vi "Export Steering Frame to VI.vi"(8 "error in (no error)":errorcluster, 10 "vi path":path, 11 "steering frame in":refnum<class "NI_Robotics_Steering Frame.lvclass">) -> (0 "error out":errorcluster, 3 "steering frame out":refnum<class "NI_Robotics_Steering Frame.lvclass">)   [LabVIEW 2017, in "NI_Robotics_Configure Steering Frame.lvlib"]
uses:
  <vilib>/robotics/Dialog/Configure Steering Frame/NI_Robotics_Configure Steering Frame.lvlib
  <vilib>/robotics/Steering/Steering Frame/NI_Robotics_Steering Frame.lvclass
  <vilib>/robotics/Utilities/Scripting/NI_Robotics_Scripting Utilities.lvlib
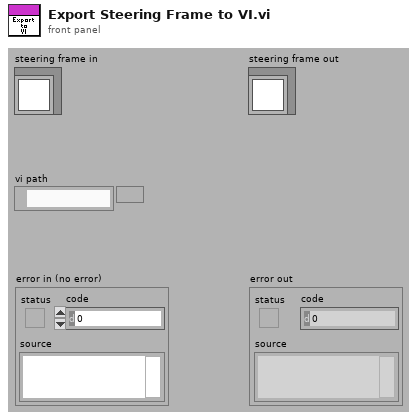
[diagram p1: front panel]
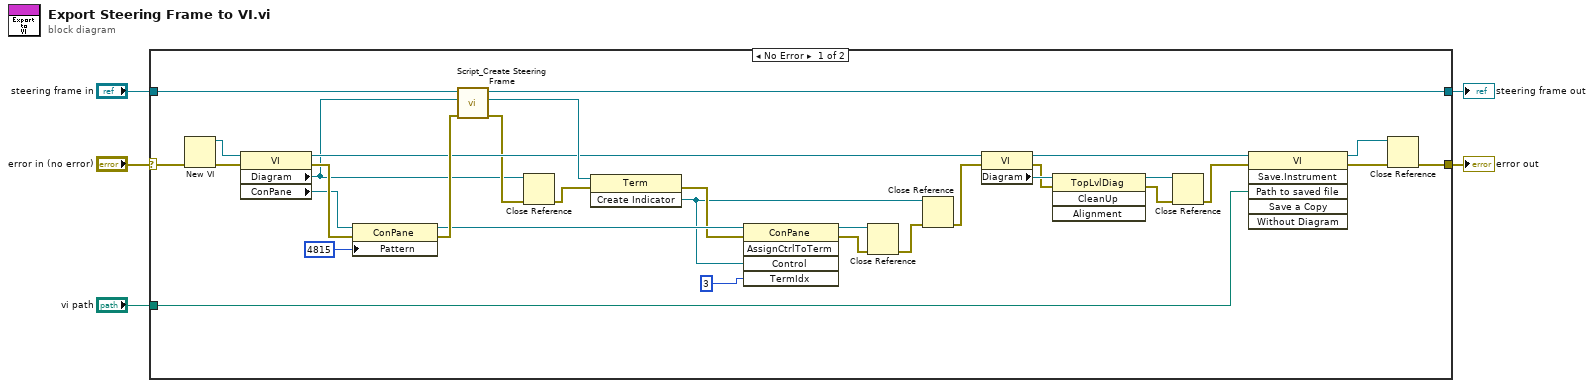
[diagram p0: block diagram]
diagram:
  n1 = case shown="No Error" "error in (no error)" {
    selector: "error in (no error)" -> [w37 w38]
    tunnel: "steering frame in" -> [w36 w39]
    tunnel: "vi path" -> [w21 _]
    tunnel: [w35 w39] -> w2
    tunnel: [w19 w38] -> w1
    frame No Error {
      n2 = New VI(8:w37) -> (0:w32:errorcluster, 3:w33:refnum<vi>)  [unwired: 6 in]
      n3 = property class="VI"(reference=w33, error in=w32) -> (reference out=w16:refnum<vi>, error out=w30:errorcluster, "Diagram"=w7:refnum<vi>, "ConPane"=w9:refnum<vi>)
      n4 = property class="ConPane"(reference=w9, error in=w30, "Pattern"=u32 4815) -> (reference out=w28:refnum<vi>, error out=w29:errorcluster)
      n5 = call <vilib>:"Script_Create Steering Frame.vi"("error in (no error)"=w29, "owner diagram refnum"=w7, "steering frame in"=w36) -> ("error out"=w8:errorcluster, "steering frame out terminal refnum"=w34:refnum<vi>, "steering frame out"=w35:refnum<class "NI_Robotics_Steering Frame.lvclass">)  [unwired: 4 in, 2 out]
      n6 = Close Reference(reference=w7, error in (no error)=w8) -> (error out=w6:errorcluster)
      n7 = invoke class="Term" method="Create Indicator"(reference=w34, error in=w6) -> (error out=w26:errorcluster, "Create Indicator"=w23:refnum<vi>)  [unwired: 1 in, 1 out]
      n8 = invoke class="ConPane" method="AssignCtrlToTerm"(reference=w28, error in=w26, "Control"=w23, "TermIdx"=u32 3 ("Terminal Index")) -> (reference out=w24:refnum<vi>, error out=w25:errorcluster)  [unwired: 1 in, 3 out]
      n9 = Close Reference(reference=w24, error in (no error)=w25) -> (error out=w22:errorcluster)
      n10 = Close Reference(reference=w23, error in (no error)=w22) -> (error out=w13:errorcluster)
      n11 = property class="VI"(reference=w16, error in=w13) -> (reference out=w15:refnum<vi>, error out=w14:errorcluster, "Diagram"=w17:refnum<vi>)
      n12 = invoke class="TopLvlDiag" method="CleanUp"(reference=w17, error in=w14) -> (reference out=w11:refnum<vi>, error out=w12:errorcluster)  [unwired: 2 in, 2 out]
      n13 = Close Reference(reference=w11, error in (no error)=w12) -> (error out=w10:errorcluster)
      n14 = invoke class="VI" method="Save.Instrument"(reference=w15, error in=w10, "Path to saved file"=w21) -> (reference out=w18:refnum<vi>, error out=w20:errorcluster)  [unwired: 3 in, 4 out]
      n15 = Close Reference(reference=w18, error in (no error)=w20) -> (error out=w19:errorcluster)
    }
    frame Error {
    }
  }
  "error out" <- w1
  "steering frame out" <- w2
